vi "ConfiguracaoCriarTask.vi"(8 "error in":errorcluster, 11 "ListaMedicaoPorta":string[][](array[string])) -> (0 "error out":errorcluster, 3 "AnalogTasks":cluster{"Function":i32, "Task":refnum<k21>}[](array[cluster]))   [LabVIEW 2019]
uses:
  bad46583-adc6-4985-aa6e-4532668e77c6.vi
  <vilib>/Array/Sort 2D Array - Pop Stack.vi
  <vilib>/Array/Sort 2D Array - Push Stack.vi
  VariaveisTaskMedicao.vi
panel:
  out "AnalogTasks":string[][](array[string])
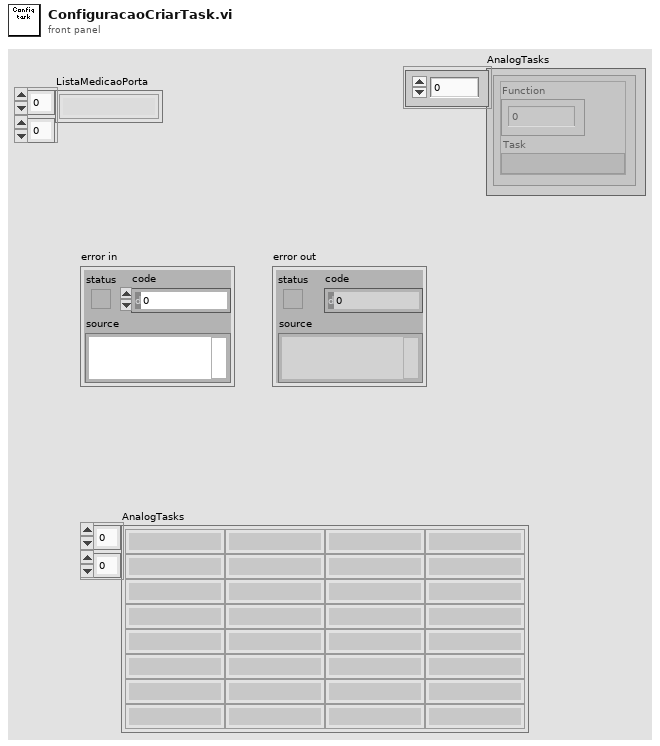
[diagram p1: front panel]
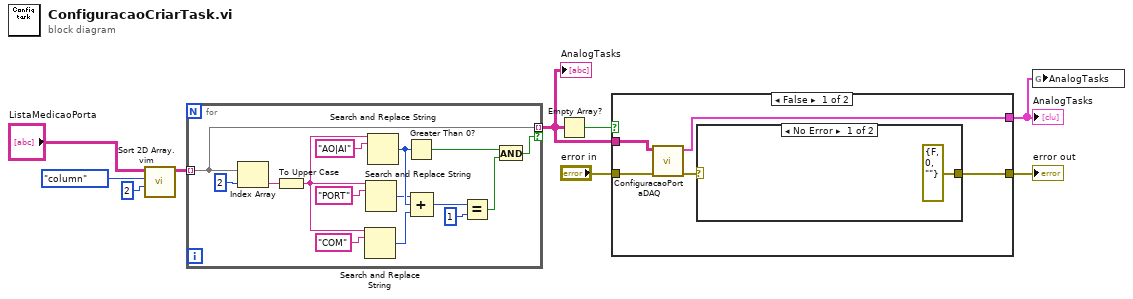
[diagram p0: block diagram]
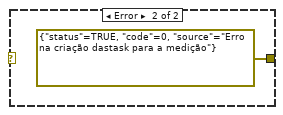
[diagram p2: hidden frame]
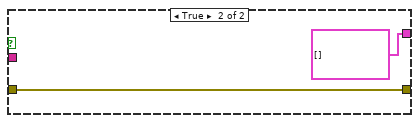
[diagram p3: hidden frame]
diagram:
  n1 = call "Sort 2D Array.vim"("index"=2, "dimension to index (column)"=enum16{"column", "row"}."column", "2D array"="ListaMedicaoPorta") -> ("sorted 2D array"=w5:string[][])  [unwired: 7 in, 1 out]
  n2 = for {
    tunnel: w5 -> [w12] mode=indexing
    tunnel: [w12] -> w4 mode=indexing if=w11
    n3 = Index Array(array=w12, index=2) -> (element=w23:string)
    n4 = To Upper Case(1:w23) -> (0:w10:string)
    n5 = Search and Replace String(input string=w10, search string="COM") -> (number of replacements=w19:i32)  [unwired: 6 in, 3 out]
    n6 = Search and Replace String(input string=w10, search string="PORT") -> (number of replacements=w17:i32)  [unwired: 6 in, 3 out]
    n7 = Search and Replace String(input string=w10, search string="AO|AI") -> (number of replacements=w18:i32)  [unwired: 6 in, 3 out]
    n8 = Greater Than 0?(x=w18) -> (x > 0?=w14:bool)
    n9 = Compound Arithmetic op=ADD(w17, w18, w19) -> (w16:i32)
    n10 = Equal?(x=w16, y=1) -> (x = y?=w13:bool)
    n11 = And(x=w14, y=w13) -> (x .and. y?=w11:bool)
  }
  "AnalogTasks" <- w4
  n12 = Empty Array?(array=w4) -> (empty?=w3:bool)
  n13 = case shown="False" w3 {
    tunnel: "error in" -> [w28 w33]
    tunnel: [w29 w33] -> w6
    tunnel: w4 -> [w26 _]
    tunnel: [w25 cluster{"Function":i32, "Task":refnum<k21>}[] [] ("AnalogTasks")] -> w2
    frame False {
      n14 = call "ConfiguracaoPortaDAQ.vi"("error in"=w28, "AnalogTasksConfiguration"=w26) -> ("error out"=w27:errorcluster, "AnalogTasks"=w25:cluster{"Function":i32, "Task":refnum<k21>}[])  [unwired: 7 in, 1 out]
      n15 = case shown="No Error" w27 {
        tunnel: [errorcluster {"status"=FALSE, "code"=0, "source"=""} ("error IO") errorcluster {"status"=TRUE, "code"=0, "source"="Erro na criação dastask para a medição"} ("error IO")] -> w29
        frame No Error {
        }
        frame Error {
        }
      }
    }
    frame True {
    }
  }
  "error out" <- w6
  "AnalogTasks" <- w2
  n16 = global write "VariaveisTaskMedicao.vi" "AnalogTasks"(w2) -> ()
